vi "Parse VI Name from Call Chain.vi"(11 "call chain":string[](array[string])) -> (3 "VI Name":string)   [LabVIEW 2020, in "LMock Mock.lvclass"]
uses:
  LMock Mock.lvclass
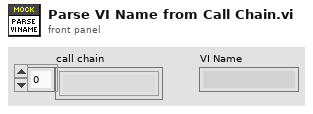
[diagram p1: front panel]
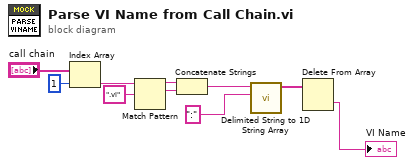
[diagram p0: block diagram]
diagram:
  n1 = Index Array(array="call chain", index=1) -> (element=w6:string)
  n2 = Match Pattern(string=w6, regular expression=".vi") -> (before substring=w4:string, match substring=w5:string)  [unwired: 1 in, 2 out]
  n3 = Concatenate Strings(w4, w5) -> (w7:string)
  n4 = call <vilib>:"Delimited String to 1D String Array.vi"("delimiter"=":", "delimited string"=w7) -> ("string array"=w9:string[])  [unwired: 9 in]
  n5 = Delete From Array(array=w9) -> (deleted portion=→"VI Name":string)  [unwired: 2 in, 1 out]
